vi "Overlay_Lichtgitterposition _Livebild.vi"(8 "error in":errorcluster, 9 "gerade?":bool, 10 "Image in":T6, 11 "Cluster in":T1={"Initialisierung"={"Online?"=FALSE, "Grundpfad"=path "", "Kamera Oben"="", "IP-Adresse Flüssiglinse"="", "Flüssiglinse"=refnum, "Kamera Unten"="", "IP-Adresse SPS"="", "SPS-Verbindung"={"TCP Connection Ref"=refnum, "IP address"="", "timeout ms"=5000, "Connected?"=FALSE, "PLC Type"=enum."S7 1200", "Rack S7 400"=0, "Slot S7 400"=0, "PDU Size"=0, "connection semaphore"=refnum}, "IP-Adresse Lichtgitter"="", "Lichtgitter"=refnum, "Skalierungsfaktor"=0.0, "Bilder Oben"=[], "Bild Unten"=refnum, "Bild Ausschnitt Unten"=refnum}, "Einstellungen"={"Gesamtablauf gestartet"=FALSE, "i. O. Bilder speichern"=FALSE, "Bildspeicherung Offline"=FALSE, "Ausgewähltes Offline-Datum"="", "Ausgewähltes Offline-Teil"="", "Speicherpfad Bilder"=path ""}, "Artikeldaten"={"Artikelnummer"="", "Fertigungsauftrag"="", "Muster ISO"=refnum, "Belichtungszeit Referenzmarken"=0.0, "Fokus Referenzmarken"=0.0, "Belichtungszeit ISO"=0.0, "Fokus ISO"=0.0, "Belichtungszeit Unten"=0.0, "Kontaktanzahl"=0, "Aktueller Kontakt"=0, "Kontaktposition"={"x"=0.0, "y"=0.0}, "Winkel ISO"=0.0, "ISO-Muster nicht vorhanden"=FALSE}, "Werte Kamera Oben"={"Koordinatensystem"={"Punkt x-Achse"={"X"=0.0, "Y"=0.0}, "Ursprung"={"X"=0.0, "Y"=0.0}, "Punkt y-Achse"={"X"=0.0, "Y"=0.0}}, "Position Kontakt"={"x"=0.0, "y"=0.0}, "Winkel Kontakt"=0.0}, "Werte Kamera Unten"={"Prüfung Unten n. i. O."=FALSE}, "Werte Lichtgitter"={"Messwerte Referenzmarken"=[], "Mittelpunkt Referenzmarken"={"x"=0.0, "y"=0.0}, "Messwerte Kontakt"=[], "Offset"={"x"=0.0, "y"=0.0}}, "Rückmeldungen"={"Koordinaten ermittelt"=FALSE, "Vermessung Lichtgitter fertig"=FALSE, "Nachkontrolle Kamera Unten fertig"=FALSE}, "Fehler"={"Referenzen nicht gefunden"=FALSE, "Kontakt nicht gefunden"=FALSE, "Referenzen nicht in Lichtgitter"=FALSE, "Kontakt zu groß"=FALSE, "Kontakt zu klein"=FALSE}, "Statistik"={"Statistiken"=[]}, "Timer"={"Timer Start Position"=0, "Timer Start Lichtgitter"=0, "Timer Start Kamera Unten"=0}}) -> (0 "error out":errorcluster, 2 "Image out":T6, 3 "Cluster out":T1={"Initialisierung"={"Online?"=FALSE, "Grundpfad"=path "", "Kamera Oben"="", "IP-Adresse Flüssiglinse"="", "Flüssiglinse"=refnum, "Kamera Unten"="", "IP-Adresse SPS"="", "SPS-Verbindung"={"TCP Connection Ref"=refnum, "IP address"="", "timeout ms"=5000, "Connected?"=FALSE, "PLC Type"=enum."S7 1200", "Rack S7 400"=0, "Slot S7 400"=0, "PDU Size"=0, "connection semaphore"=refnum}, "IP-Adresse Lichtgitter"="", "Lichtgitter"=refnum, "Skalierungsfaktor"=0.0, "Bilder Oben"=[], "Bild Unten"=refnum, "Bild Ausschnitt Unten"=refnum}, "Einstellungen"={"Gesamtablauf gestartet"=FALSE, "i. O. Bilder speichern"=FALSE, "Bildspeicherung Offline"=FALSE, "Ausgewähltes Offline-Datum"="", "Ausgewähltes Offline-Teil"="", "Speicherpfad Bilder"=path ""}, "Artikeldaten"={"Artikelnummer"="", "Fertigungsauftrag"="", "Muster ISO"=refnum, "Belichtungszeit Referenzmarken"=0.0, "Fokus Referenzmarken"=0.0, "Belichtungszeit ISO"=0.0, "Fokus ISO"=0.0, "Belichtungszeit Unten"=0.0, "Kontaktanzahl"=0, "Aktueller Kontakt"=0, "Kontaktposition"={"x"=0.0, "y"=0.0}, "Winkel ISO"=0.0, "ISO-Muster nicht vorhanden"=FALSE}, "Werte Kamera Oben"={"Koordinatensystem"={"Punkt x-Achse"={"X"=0.0, "Y"=0.0}, "Ursprung"={"X"=0.0, "Y"=0.0}, "Punkt y-Achse"={"X"=0.0, "Y"=0.0}}, "Position Kontakt"={"x"=0.0, "y"=0.0}, "Winkel Kontakt"=0.0}, "Werte Kamera Unten"={"Prüfung Unten n. i. O."=FALSE}, "Werte Lichtgitter"={"Messwerte Referenzmarken"=[], "Mittelpunkt Referenzmarken"={"x"=0.0, "y"=0.0}, "Messwerte Kontakt"=[], "Offset"={"x"=0.0, "y"=0.0}}, "Rückmeldungen"={"Koordinaten ermittelt"=FALSE, "Vermessung Lichtgitter fertig"=FALSE, "Nachkontrolle Kamera Unten fertig"=FALSE}, "Fehler"={"Referenzen nicht gefunden"=FALSE, "Kontakt nicht gefunden"=FALSE, "Referenzen nicht in Lichtgitter"=FALSE, "Kontakt zu groß"=FALSE, "Kontakt zu klein"=FALSE}, "Statistik"={"Statistiken"=[]}, "Timer"={"Timer Start Position"=0, "Timer Start Lichtgitter"=0, "Timer Start Kamera Unten"=0}})   [LabVIEW 2024]
uses:
  Cluster.ctl
  Kontaktmontagemodul.exe/1abvi3w/vi.lib/userDefined/High Color/IMAQdx.ctl
  Kontaktmontagemodul.exe/1abvi3w/vi.lib/DATA AHEAD/SP7/typedefs/S7 Connection.ctl
  Kontaktmontagemodul.exe/1abvi3w/vi.lib/DATA AHEAD/SP7/typedefs/PLC Type.ctl
  Kontaktmontagemodul.exe/1abvi3w/vi.lib/vision/Image Controls.llb/IMAQ Image.ctl
  Koordinatensystem.ctl
  Statistik.ctl
  Kontaktmontagemodul.exe/1abvi3w/vi.lib/Analysis/Matrix/Datatypes/RealMatrix.ctl
  Kontaktmontagemodul.exe/1abvi3w/vi.lib/vision/NI_Vision_Development_Module.lvlib
  Kontaktmontagemodul.exe/1abvi3w/vi.lib/Analysis/Matrix/NI_Matrix.lvlib
  Kontaktmontagemodul.exe/1abvi3w/vi.lib/DATA AHEAD/SP7/SP7.lvlib
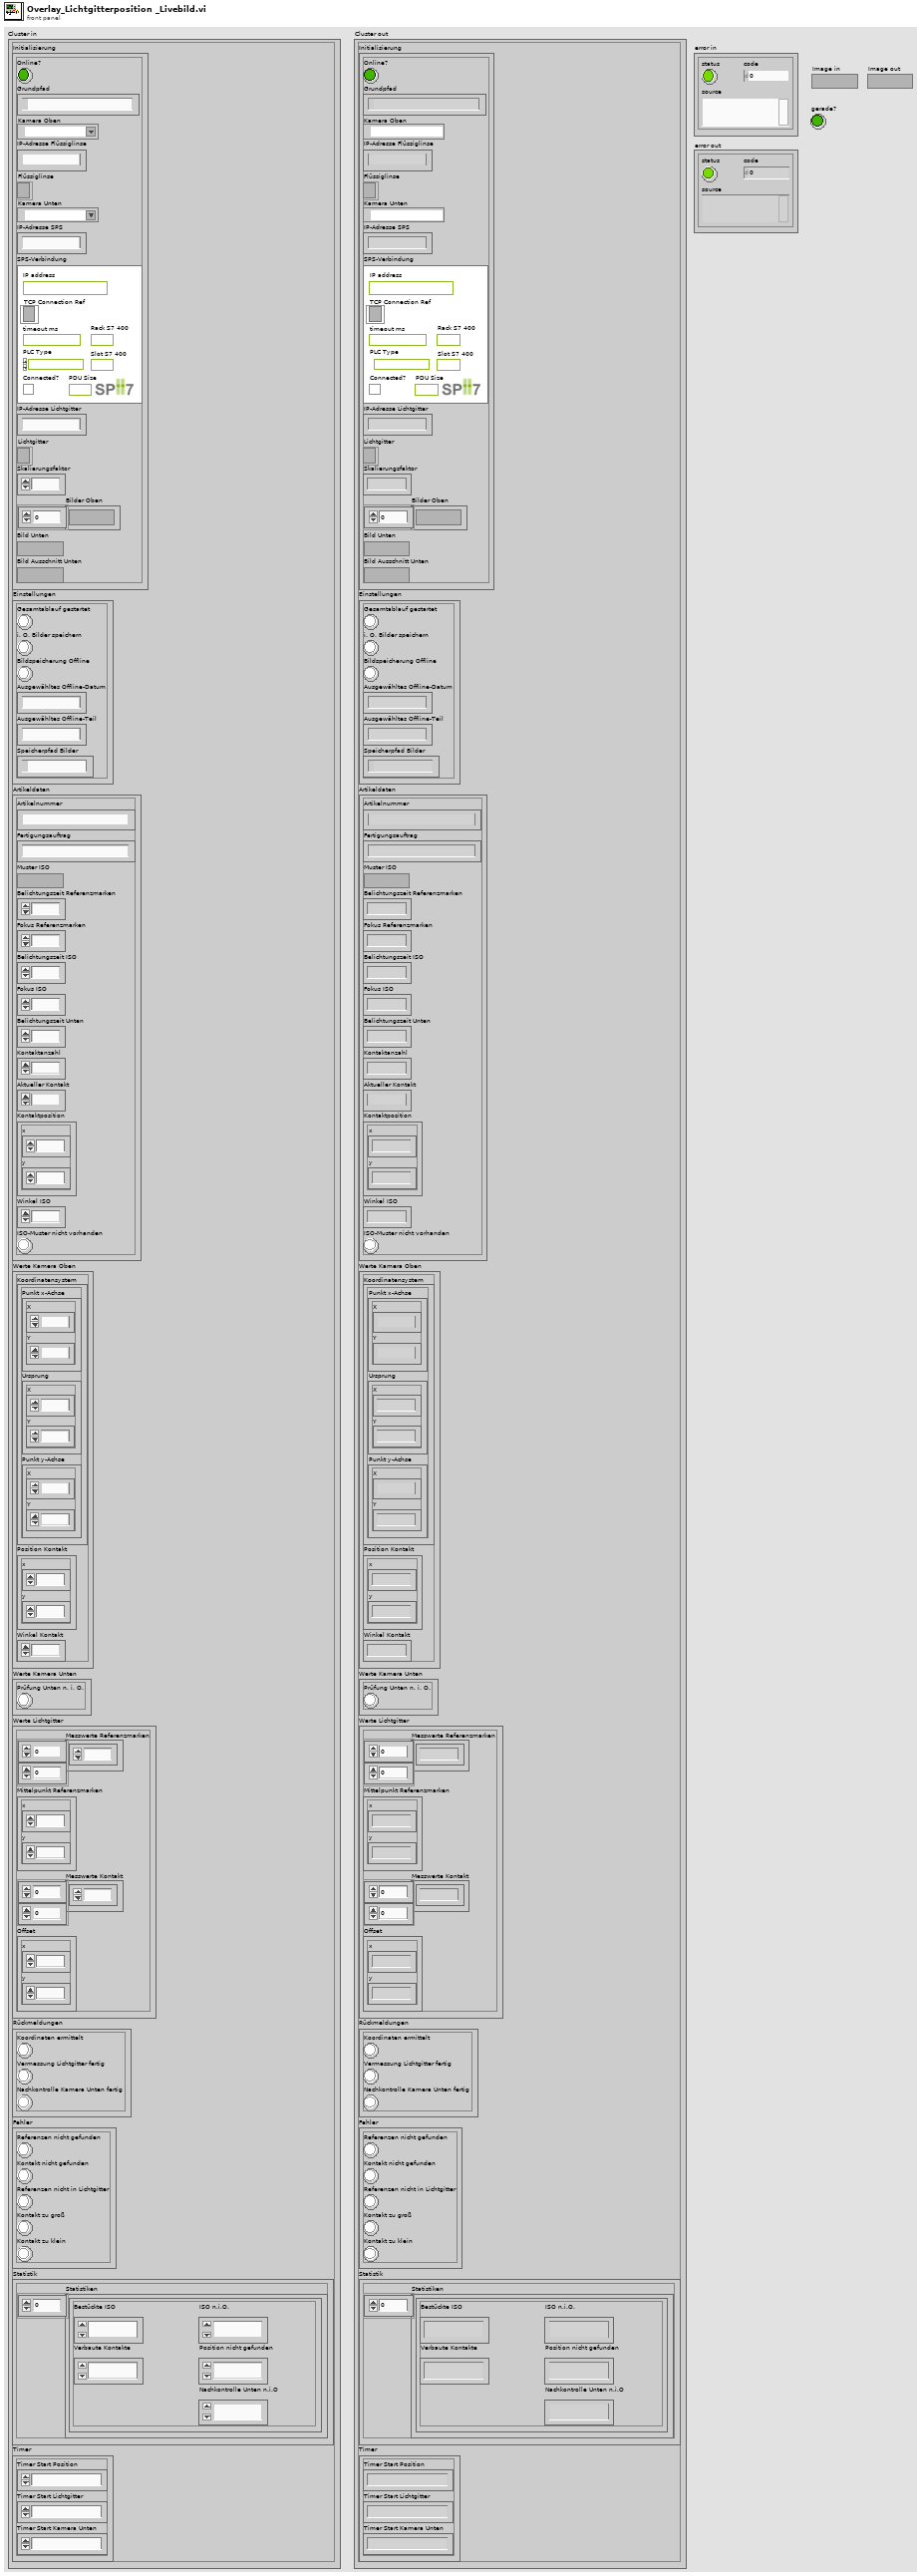
[diagram p1: front panel]
types:
  T1 = typedef "Cluster.ctl" = cluster{"Initialisierung":cluster{"Online?":bool, "Grundpfad":path, "Kamera Oben":T2, "IP-Adresse Flüssiglinse":string, "Flüssiglinse":refnum<k5>, "Kamera Unten":T2, "IP-Adresse SPS":string, "SPS-Verbindung":T3, "IP-Adresse Lichtgitter":string, "Lichtgitter":refnum<k5>, "Skalierungsfaktor":dbl, "Bilder Oben":T6[], "Bild Unten":T6, "Bild Ausschnitt Unten":T6}, "Einstellungen":cluster{"Gesamtablauf gestartet":bool, "i. O. Bilder speichern":bool, "Bildspeicherung Offline":bool, "Ausgewähltes Offline-Datum":string, "Ausgewähltes Offline-Teil":string, "Speicherpfad Bilder":path}, "Artikeldaten":cluster{"Artikelnummer":string, "Fertigungsauftrag":string, "Muster ISO":T6, "Belichtungszeit Referenzmarken":dbl, "Fokus Referenzmarken":dbl, "Belichtungszeit ISO":dbl, "Fokus ISO":dbl, "Belichtungszeit Unten":dbl, "Kontaktanzahl":u32, "Aktueller Kontakt":i16, "Kontaktposition":cluster{"x":sgl, "y":sgl}, "Winkel ISO":sgl, "ISO-Muster nicht vorhanden":bool}, "Werte Kamera Oben":cluster{"Koordinatensystem":T7, "Position Kontakt":cluster{"x":dbl, "y":dbl}, "Winkel Kontakt":dbl}, "Werte Kamera Unten":cluster{"Prüfung Unten n. i. O.":bool}, "Werte Lichtgitter":cluster{"Messwerte Referenzmarken":dbl[][], "Mittelpunkt Referenzmarken":cluster{"x":dbl, "y":dbl}, "Messwerte Kontakt":dbl[][], "Offset":cluster{"x":dbl, "y":dbl}}, "Rückmeldungen":cluster{"Koordinaten ermittelt":bool, "Vermessung Lichtgitter fertig":bool, "Nachkontrolle Kamera Unten fertig":bool}, "Fehler":cluster{"Referenzen nicht gefunden":bool, "Kontakt nicht gefunden":bool, "Referenzen nicht in Lichtgitter":bool, "Kontakt zu groß":bool, "Kontakt zu klein":bool}, "Statistik":cluster{"Statistiken":T8[]}, "Timer":cluster{"Timer Start Position":u32, "Timer Start Lichtgitter":u32, "Timer Start Kamera Unten":u32}}
  T2 = typedef "IMAQdx.ctl" = refnum<k21>
  T3 = typedef "SP7.lvlib/S7 Connection.ctl" = cluster{"TCP Connection Ref":refnum<k5>, "IP address":string, "timeout ms":i32, "Connected?":bool, "PLC Type":T4, "Rack S7 400":u8, "Slot S7 400":u8, "PDU Size":u16, "connection semaphore":T5}
  T4 = typedef "SP7.lvlib/PLC Type.ctl" = enum16{"S7 200", "S7 300/400", "S7 1200", "S7 1500", "LOGO!8"}
  T5 = typedef "Semaphore RefNum" = refnum<k1>
  T6 = typedef "IMAQ Image.ctl" = refnum<image>
  T7 = typedef "Koordinatensystem.ctl" = cluster{"Punkt x-Achse":cluster{"X":sgl, "Y":sgl}, "Ursprung":cluster{"X":sgl, "Y":sgl}, "Punkt y-Achse":cluster{"X":sgl, "Y":sgl}}
  T8 = typedef "Statistik.ctl" = cluster{"Bestückte ISO":u32, "Verbaute Kontakte":u32, "ISO n.i.O.":u32, "Nachkontrolle Unten n.i.O":u32, "Position nicht gefunden":u32}
  T9 = typedef "NI_Matrix.lvlib/RealMatrix.ctl" = dbl[][]
  T10 = cluster{"Farbe Kreis":u32, "Kreis ausfüllen?":bool, "Bounding Rechteck anzeigen?":bool, "Farbe Bounding Rechteck":u32}
  T11 = cluster{"Position":cluster{"X":sgl, "Y":sgl}, "Radius":dbl, "Score":dbl}
  T12 = cluster{"Position":cluster{"X":sgl, "Y":sgl}, "Radius":dbl, "Score":dbl}[]
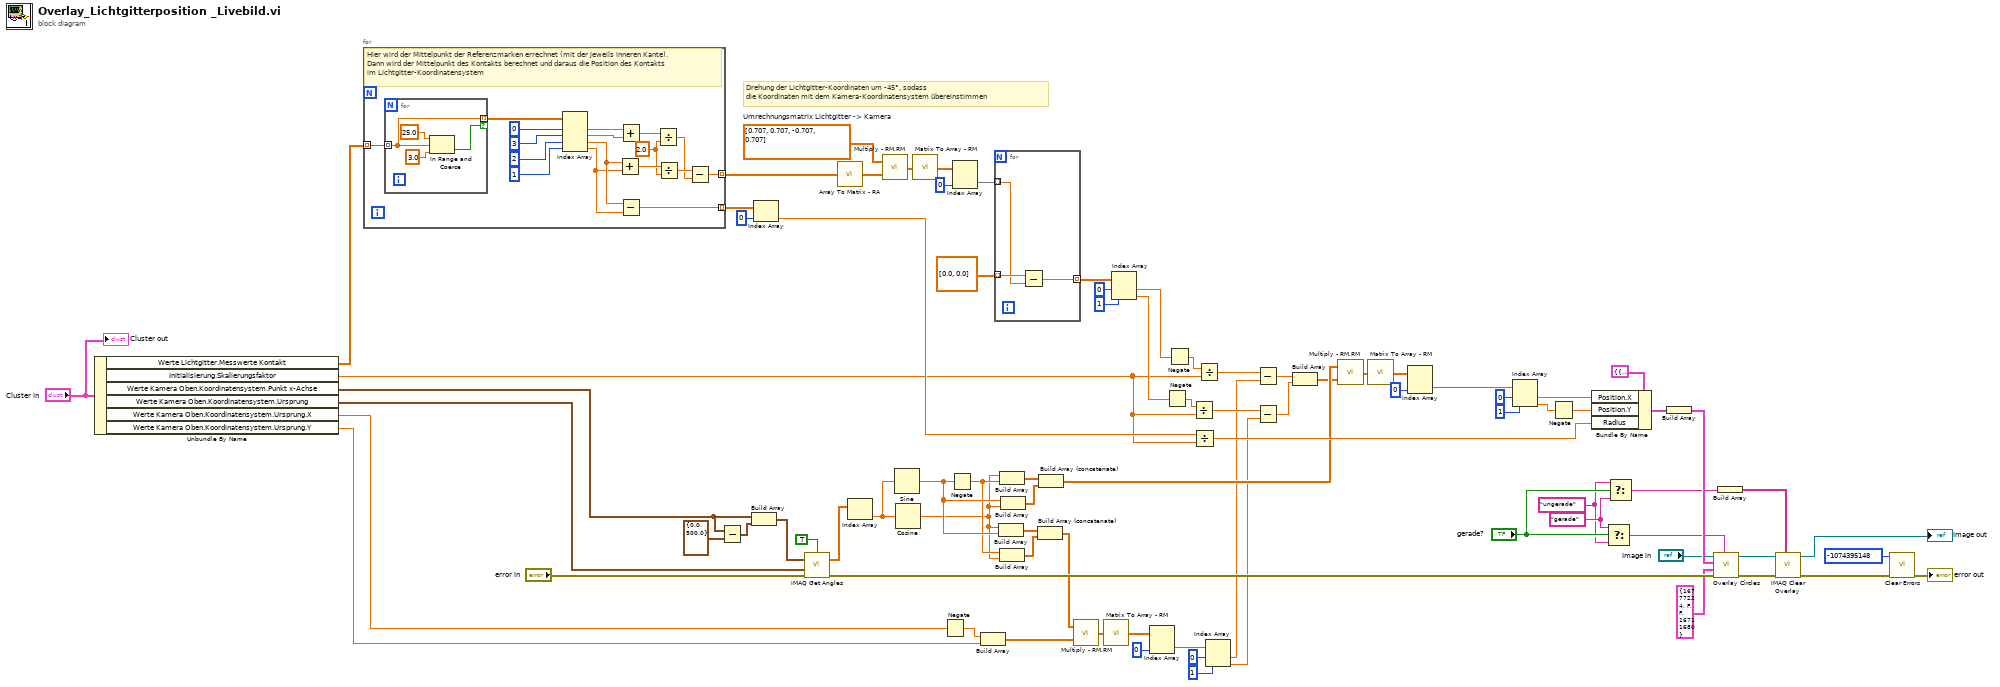
[diagram p0: block diagram]
diagram:
  w5 = "ungerade" ("Group")
  w6 = "gerade" ("Group")
  w68 = T9 [[0.707, 0.707], [-0.707, 0.707]]  # Umrechnungsmatrix Lichtgitter -> Kamera
  # "Drehung der Lichtgitter-Koordinaten um -45°, sodass\ndie Koordinaten mit dem Kamera-Koordinatensystem übereinstimmen"
  n1 = Unbundle By Name("Cluster in") -> ("Werte Lichtgitter.Messwerte Kontakt"=w55:dbl[][], "Initialisierung.Skalierungsfaktor"=w1:dbl, "Werte Kamera Oben.Koordinatensystem.Punkt x-Achse"=w56:cluster{"X":sgl, "Y":sgl}, "Werte Kamera Oben.Koordinatensystem.Ursprung"=w57:cluster{"X":sgl, "Y":sgl}, "Werte Kamera Oben.Koordinatensystem.Ursprung.X"=w36:sgl, "Werte Kamera Oben.Koordinatensystem.Ursprung.Y"=w35:sgl)
  n2 = for {
    tunnel: w55 -> [w91] mode=indexing
    tunnel: [w101] -> w69 mode=indexing
    tunnel: [w87] -> w60 mode=indexing
    w92 = 2.0 ("y")
    # "Hier wird der Mittelpunkt der Referenzmarken errechnet (mit der jeweils inneren Kante). Dann wird der Mittelpunkt des Kontakts berechnet und daraus die Position des Kontakts im Lichtgitter-Koordinatensystem"
    n3 = for {
      tunnel: w91 -> [w103] mode=indexing
      tunnel: [w103] -> w90 mode=indexing if=w102
      n4 = In Range and Coerce(upper limit=25.0, x=w103, lower limit=3.0) -> (In Range?=w102:bool)  [unwired: 1 out]
    }
    n5 = Index Array(array=w90, index #1=0 ("index"), index #2=3 ("index"), index #3=2 ("index"), index #4=1 ("index")) -> (element #1=w94:dbl, element #2=w93:dbl, element #3=w89:dbl, element #4=w88:dbl)
    n6 = Add(x=w89, y=w88) -> (x+y=w99:dbl)
    n7 = Add(x=w94, y=w93) -> (x+y=w100:dbl)
    n8 = Subtract(x=w89, y=w88) -> (x-y=w87:dbl)
    n9 = Divide(x=w100, y=w92) -> (x/y=w85:dbl)
    n10 = Divide(x=w99, y=w92) -> (x/y=w86:dbl)
    n11 = Subtract(x=w86, y=w85) -> (x-y=w101:dbl)
  }
  n12 = Subtract(x=w56, y=cluster{"X":sgl, "Y":sgl} {"X"=0.0, "Y"=500.0}) -> (x-y=w77:cluster{"X":sgl, "Y":sgl})
  n13 = Build Array(w56, w77) -> (w76:cluster{"X":sgl, "Y":sgl}[])
  n14 = Index Array(array=w60, index=0) -> (element=w54:dbl)
  n15 = call "IMAQ Get Angles"("error in (no error)"="error in", "Vertex"=w57, "Points"=w76, "Use Vertex (No)"=TRUE) -> ("error out"=w72:errorcluster, "Angles (deg)"=w74:sgl[])  [unwired: 1 in, 1 out]
  n16 = call "Array To Matrix - RA.vi"("Real 1D Array"=w69) -> ("Real Matrix (Column Vector)"=w67:T9)
  n17 = Index Array(array=w74) -> (element=w44:sgl)  [unwired: 1 in]
  n18 = call "Multiply - RM,RM.vi"("Real Matrix B"=w67, "Real Matrix A"=w68) -> ("A * B"=w66:T9)
  n19 = Sine(x=w44) -> (sin(x)=w51:sgl)
  n20 = Cosine(x=w44) -> (cos(x)=w49:sgl)
  n21 = call "Matrix To Array - RM.vi"("Real Matrix"=w66) -> ("Real 2D Array"=w65:dbl[][])
  n22 = Negate(x=w36) -> (-x=w37:sgl)
  n23 = Negate(x=w51) -> (-x=w50:sgl)
  n24 = Index Array(array=w65, index (col)=0 ("disabled index (col)")) -> (element=w58:dbl[])  [unwired: 1 in]
  n25 = Build Array(w37, w35) -> (w33:T9)
  n26 = for {
    tunnel: w58 -> [w107] mode=indexing
    tunnel: dbl[] [0.0, 0.0] ("subarray") -> [w108] mode=indexing
    tunnel: [w106] -> w63 mode=indexing
    n27 = Subtract(x=w108, y=w107) -> (x-y=w106:dbl)
  }
  n28 = Build Array(w49, w51) -> (w48:T9)
  n29 = Build Array(w49, w50) -> (w45:T9)
  n30 = Build Array(w50, w49) -> (w47:T9)
  n31 = Build Array(w51, w49) -> (w46:T9)
  n32 = Build Array (concatenate)(w48, w47) -> (w34:T9)
  n33 = Build Array (concatenate)(w45, w46) -> (w20:T9)
  n34 = call "Multiply - RM,RM.vi"("Real Matrix B"=w33, "Real Matrix A"=w34) -> ("A * B"=w39:T9)
  n35 = call "Matrix To Array - RM.vi"("Real Matrix"=w39) -> ("Real 2D Array"=w40:dbl[][])
  n36 = Index Array(array=w63, index #1=0 ("index"), index #2=1 ("index")) -> (element #1=w21:dbl, element #2=w22:dbl)
  n37 = Index Array(array=w40, index (col)=0 ("disabled index (col)")) -> (element=w43:dbl[])  [unwired: 1 in]
  n38 = Negate(x=w22) -> (-x=w23:dbl)
  n39 = Negate(x=w21) -> (-x=w24:dbl)
  n40 = Divide(x=w23, y=w1) -> (x/y=w18:dbl)
  n41 = Divide(x=w54, y=w1) -> (x/y=w25:dbl)
  n42 = Divide(x=w24, y=w1) -> (x/y=w19:dbl)
  n43 = Index Array(array=w43, index #1=0 ("index"), index #2=1 ("index")) -> (element #1=w17:dbl, element #2=w16:dbl)
  n44 = Subtract(x=w19, y=w17) -> (x-y=w32:dbl)
  n45 = Subtract(x=w18, y=w16) -> (x-y=w15:dbl)
  n46 = Build Array(w32, w15) -> (w14:T9)
  n47 = call "Multiply - RM,RM.vi"("Real Matrix B"=w14, "Real Matrix A"=w20) -> ("A * B"=w79:T9)
  n48 = call "Matrix To Array - RM.vi"("Real Matrix"=w79) -> ("Real 2D Array"=w80:dbl[][])
  n49 = Index Array(array=w80, index (col)=0 ("disabled index (col)")) -> (element=w28:dbl[])  [unwired: 1 in]
  n50 = Index Array(array=w28, index #1=0 ("index"), index #2=1 ("index")) -> (element #1=w26:dbl, element #2=w31:dbl)
  n51 = Negate(x=w31) -> (-x=w27:dbl)
  n52 = Bundle By Name(cluster=T11 {"Position"={"X"=0.0, "Y"=0.0}, "Radius"=0.0, "Score"=0.0} ("Circle Descriptor"), "Position.X"=w26, "Position.Y"=w27, "Radius"=w25) -> (w83:T11)
  n53 = Select(t=w6, s="gerade?", f=w5) -> (s? t:f=w10:string)
  n54 = Select(t=w5, s="gerade?", f=w6) -> (s? t:f=w8:string)
  n55 = Build Array(w83) -> (w71:T12)
  n56 = call "Overlay Circles.vi"("Group"=w10, "error in"=w72, "Einstellungen"=T10 {"Farbe Kreis"=16777224, "Kreis ausfüllen?"=FALSE, "Bounding Rechteck anzeigen?"=FALSE, "Farbe Bounding Rechteck"=16711680}, "Circles"=w71, "Image in"="Image in") -> ("error out"=w13:errorcluster, "Image out"=w12:T6)  [unwired: 5 in]
  n57 = Build Array(w8) -> (w7:string[])
  n58 = call "IMAQ Clear Overlay"("Groups"=w7, "error in (no error)"=w13, "Image"=w12) -> ("error out"=w4:errorcluster, "Image Out"=→"Image out":T6)  [unwired: 7 in]
  n59 = call "Clear Errors.vi"("error in (no error)"=w4, "specific error code to clear (0: all)"=-1074395148) -> ("error out"=→"error out":errorcluster)  [unwired: 4 in, 1 out]
  "Cluster out" <- "Cluster in"
